vi "IMU Loop.vi"() -> ()   [LabVIEW 2012]
panel:
  in  "stop?":bool
  in  "error in":errorcluster
  out "error out 2":errorcluster
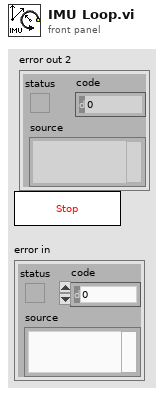
[diagram p1: front panel]
types:
  T1 = enum16{"Husky", "Galatea", "Sim Husky", "Sim Galatea"}
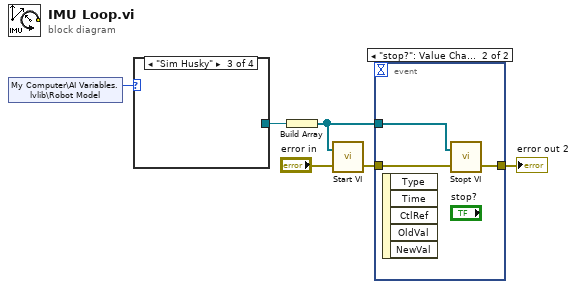
[diagram p0: block diagram]
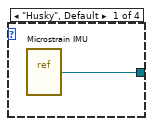
[diagram p2: hidden frame]
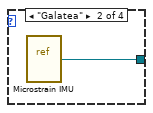
[diagram p3: hidden frame]
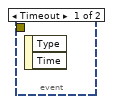
[diagram p5: hidden frame]
diagram:
  n1 = shared-variable "My Computer\\AI Variables.lvlib\\Robot Model"() -> (w2:T1)  [unwired: 1 in, 1 out]
  n2 = case shown="\"Sim Husky\"" w2 {
    tunnel: [w7 w8 _ _] -> w1
    frame "Husky", Default {
      n3 = vi-ref "Microstrain IMU.vi"() -> (w7:refnum<vi>)
    }
    frame "Galatea" {
      n4 = vi-ref "Microstrain IMU.vi"() -> (w8:refnum<vi>)
    }
    frame "Sim Husky" {
    }
    frame "Sim Galatea" {
    }
  }
  n5 = Build Array(w1) -> (w6:refnum<vi>[])
  n6 = call "Start VI.vi"("error in"="error in", "VI refnum"=w6) -> ("error out"=w4:errorcluster)  [unwired: 1 in]
  n7 = event shown="[1] \"stop?\": Value Change" {
    selector: _ -> [_ _]
    dyn-events: _ -> [_ _]
    timeout: _ -> [_ _]
    tunnel: w6 -> [_ w11]
    tunnel: [_ w10] -> w5
    tunnel: w4 -> [_ w9]
    event Timeout {
      n8 = event-data() -> ()  [unwired: 1 in, 2 out]
    }
    event "stop?": Value Change {
      n9 = event-data() -> ()  [unwired: 1 in, 5 out]
      n10 = call "Stopt VI.vi"("error in"=w9, "VI refnum"=w11) -> ("error out"=w10:errorcluster)  [unwired: 1 in]
    }
  }
  "error out 2" <- w5
